vi "Example 8 - For Loops.vi"() -> ()   [LabVIEW 2015]
uses:
  library/Loop Terminal Type.ctl
  library/Scripting.lvlib
panel:
  in  "Stop Condition?":bool=TRUE
  in  "Number of Static Parallel Instances":i32
  in  "Loop Count?":bool=TRUE
  in  "Loop Terminal Types":T1[](array[typedef])
  in  "Conditional Terminal?":bool=TRUE
  in  "Inputs Indexing?":bool[](array[boolean])=[TRUE, TRUE]
  in  "Shift Registers?":bool=TRUE
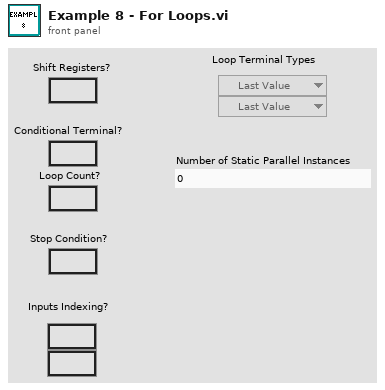
[diagram p1: front panel]
types:
  T1 = typedef "Scripting.lvlib/Loop Terminal Type.ctl" = enum16{"Last Value", "Indexing", "Concatenating"}
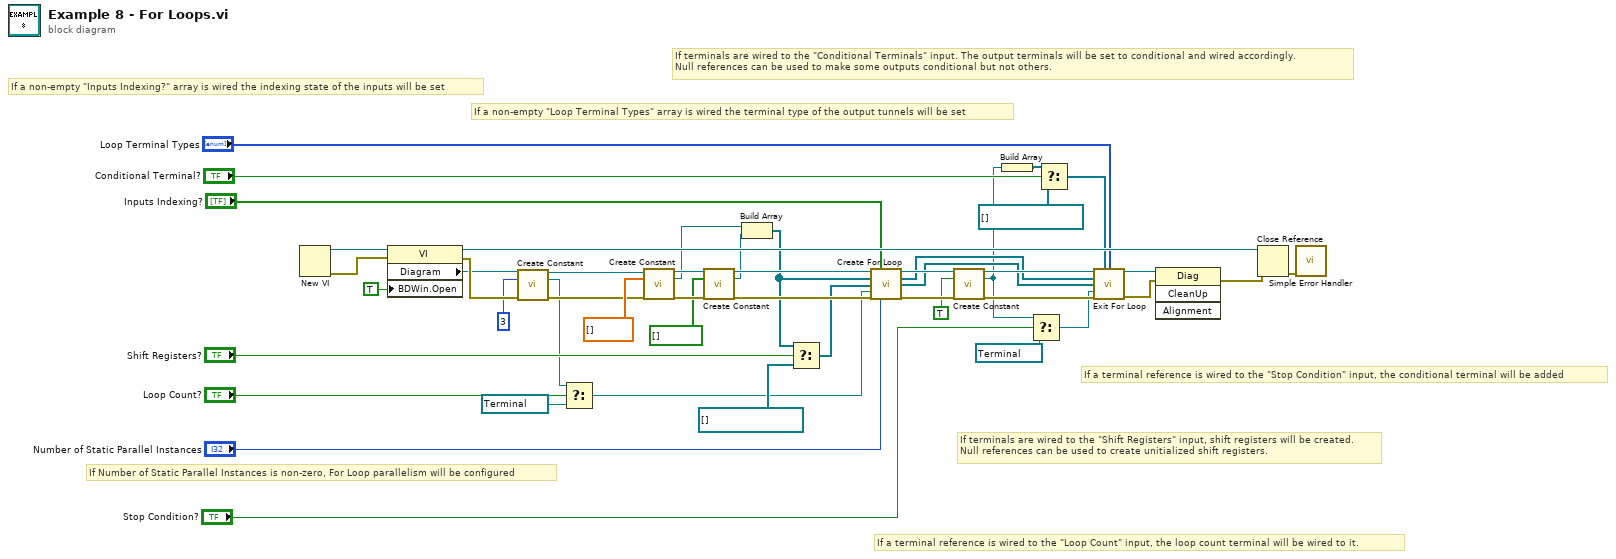
[diagram p0: block diagram]
diagram:
  # "If a terminal reference is wired to the \"Stop Condition\" input, the conditional terminal will be added"
  # "If Number of Static Parallel Instances is non-zero, For Loop parallelism will be configured"
  # "If a terminal reference is wired to the \"Loop Count\" input, the loop count terminal will be wired to it."
  # "If terminals are wired to the \"Conditional Terminals\" input. The output terminals will be set to conditional and wired accordingly.\nNull references can be used to make some outputs conditional but not others."
  # "If a non-empty \"Inputs Indexing?\" array is wired the indexing state of the inputs will be set"
  # "If terminals are wired to the \"Shift Registers\" input, shift registers will be created.\nNull references can be used to create unitialized shift registers."
  # "If a non-empty \"Loop Terminal Types\" array is wired the terminal type of the output tunnels will be set"
  n1 = New VI() -> (0:w29:errorcluster, 3:w30:refnum<vi>)  [unwired: 7 in]
  n2 = property class="VI"(reference=w30, error in=w29, "BDWin.Open"=TRUE ("Block Diagram Window:Open")) -> (reference out=w45:refnum<vi>, error out=w43:errorcluster, "Diagram"=w12:refnum<vi>)
  n3 = call "Create Constant.vi"("Diagram in"=w12, "Type"=3, "error in (no error)"=w43) -> ("Diagram out"=w11:refnum<vi>, "Terminal"=w8:refnum<vi>, "error out"=w13:errorcluster)  [unwired: 10 in]
  n4 = Select(t=w8, s="Loop Count?", f=refnum<vi> refnum) -> (s? t:f=w6:refnum<vi>)
  n5 = call "Create Constant.vi"("Diagram in"=w11, "Type"=dbl[] [], "error in (no error)"=w13) -> ("Diagram out"=w44:refnum<vi>, "Terminal"=w39:refnum<vi>, "error out"=w42:errorcluster)  [unwired: 10 in]
  n6 = call "Create Constant.vi"("Diagram in"=w44, "Type"=bool[] [], "error in (no error)"=w42) -> ("Diagram out"=w41:refnum<vi>, "Terminal"=w38:refnum<vi>, "error out"=w40:errorcluster)  [unwired: 10 in]
  n7 = Build Array(w39, w38) -> (w28:refnum<vi>[])
  n8 = Select(t=w28, s="Shift Registers?", f=refnum<vi>[] []) -> (s? t:f=w26:refnum<vi>[])
  n9 = call "Create For Loop.vi"("Diagram in"=w41, "Inputs Indexing?"="Inputs Indexing?", "Inputs"=w28, "Shift Register Inputs"=w26, "Loop Count Terminal"=w6, "error in (no error)"=w40, "Number of Static Parallel Instances"="Number of Static Parallel Instances") -> ("Diagram out"=w37:refnum<vi>, "Inputs"=w33:refnum<vi>[], "Shift Registers"=w22:refnum<vi>[], "error out"=w36:errorcluster)  [unwired: 4 in, 1 out]
  n10 = call "Create Constant.vi"("Diagram in"=w37, "Type"=TRUE, "error in (no error)"=w36) -> ("Diagram out"=w34:refnum<vi>, "Terminal"=w3:refnum<vi>, "error out"=w32:errorcluster)  [unwired: 10 in]
  n11 = Build Array(w3) -> (w17:refnum<vi>[])
  n12 = Select(t=w3, s="Stop Condition?", f=refnum<vi> refnum) -> (s? t:f=w1:refnum<vi>)
  n13 = Select(t=w17, s="Conditional Terminal?", f=refnum<vi>[] []) -> (s? t:f=w15:refnum<vi>[])
  n14 = call "Exit For Loop.vi"("Diagram in"=w34, "Conditional Terminals"=w15, "Loop Terminal Types"="Loop Terminal Types", "Outputs"=w33, "Shift Registers"=w22, "Stop Condition"=w1, "error in (no error)"=w32) -> ("Diagram out"=w24:refnum<vi>, "error out"=w23:errorcluster)  [unwired: 5 in, 2 out]
  n15 = invoke class="Diag" method="CleanUp"(reference=w24, error in=w23) -> (error out=w31:errorcluster)  [unwired: 2 in, 3 out]
  n16 = Close Reference(reference=w45, error in (no error)=w31) -> (error out=w46:errorcluster)
  n17 = call <vilib>:"Simple Error Handler.vi"("error in (no error)"=w46) -> ()  [unwired: 4 in, 5 out]
